vi "WILT.vi"() -> ()   [LabVIEW 2016] (continued)
        n1516 = call "WILT Station Controller.vi"("Station Number"=w3052, "GUI Aisle in"=w3054, "Drying Time (Min)"=w3037, "Current Threshold"=w3042, "Station Test State In"=w3047, "Error In"=w3051, "Aisle Location Index"=w3049, "Cool Down Period (seconds)"=w3038, "Disable Flood Check"=w3032, "Delay After Cutout (sec)"=w3034, "Previous Run Statistics"=w3036, "Send Restart Every? (Sec)"=w3039, "Agilent Valve and Switch Locations"=w3043, "Injection Times"=w3044, "Enable Start Retry"=w3041, "Day/Night Cycle"=w3045, "Final Start Presses"=w3033, "Semaphore"=w3035) -> ("GUI Aisle 1"=w3053:T3[], "Test Station Out"=w3048:T7, "Enable Start Retry Out"=w3040:bool[], "Error Out"=w3050:errorcluster)  [unwired: 5 in, 1 out]
        n1517 = Bundle By Name(cluster=w3056, "GUI Aisle 1 (SLAT)."=w3053, "Station Test State Cluster"=w3048, "Enable Start Retry Array"=w3040) -> (w3055:T24)
        n1518 = call <vilib>:"Add State(s) to Queue__jki_lib_state_machine.vi"("State(s) in (\"\")"=w3058) -> ("States Out"=w3057:string)  [unwired: 14 in]
      }
      frame "Station 12" {
        w3076 = 11  # Aisle Location Index
        w3079 = u32 12  # Station Number
        # "Control the state of station 12"
        n1519 = Unbundle By Name(w3083) -> ("Enable Start Retry Array"=w3067:bool[], "Agilent Switches"=w3069:T2[], "GUI Aisle 1 (SLAT)."=w3081:T3[], "Drying Time (Min)"=w3064:dbl[], "Current Threshold"=w3070:dbl, "Station Test State Cluster"=w3074:T7, "Station Timeout Values (1-56) Seconds"=w3065:dbl[], "Send Restart Every? (Sec)"=w3066:dbl, "Injection Times Input"=w3071:T15, "Day/Night Cycle Input"=w3072:T11)
        n1520 = local read "Previous Run Statistics"() -> (w3063:T9[])
        n1521 = local read "Delay After Cutout (Sec)"() -> (w3061:dbl)
        n1522 = local read "Final Start Presses"() -> (w3060:i32)
        n1523 = local read "Agilent Semaphore"() -> (w3062:T1[])
        n1524 = local read "Disable Flood Check"() -> (w3059:bool)
        n1525 = call "WILT Station Controller.vi"("Station Number"=w3079, "GUI Aisle in"=w3081, "Drying Time (Min)"=w3064, "Current Threshold"=w3070, "Station Test State In"=w3074, "Error In"=w3078, "Aisle Location Index"=w3076, "Cool Down Period (seconds)"=w3065, "Disable Flood Check"=w3059, "Delay After Cutout (sec)"=w3061, "Previous Run Statistics"=w3063, "Send Restart Every? (Sec)"=w3066, "Agilent Valve and Switch Locations"=w3069, "Injection Times"=w3071, "Enable Start Retry"=w3067, "Day/Night Cycle"=w3072, "Final Start Presses"=w3060, "Semaphore"=w3062) -> ("GUI Aisle 1"=w3080:T3[], "Test Station Out"=w3075:T7, "Enable Start Retry Out"=w3068:bool[], "Error Out"=w3077:errorcluster)  [unwired: 5 in, 1 out]
        n1526 = Bundle By Name(cluster=w3083, "GUI Aisle 1 (SLAT)."=w3080, "Station Test State Cluster"=w3075, "Enable Start Retry Array"=w3068) -> (w3082:T24)
        n1527 = call <vilib>:"Add State(s) to Queue__jki_lib_state_machine.vi"("State(s) in (\"\")"=w3085) -> ("States Out"=w3084:string)  [unwired: 14 in]
      }
      frame "Station 13" {
        w3104 = 0  # Aisle Location Index
        w3107 = u32 13  # Station Number
        # "Control the state of station 13"
        n1528 = Unbundle By Name(w3110) -> ("Enable Start Retry Array"=w3094:bool[], "Agilent Switches"=w3098:T2[], "GUI Aisle 1A (SLAT)."=w3108:T3[], "Drying Time (Min)"=w3091:dbl[], "Current Threshold"=w3097:dbl, "Station Test State Cluster"=w3102:T7, "Station Timeout Values (1-56) Seconds"=w3092:dbl[], "Send Restart Every? (Sec)"=w3093:dbl, "Injection Times Input"=w3099:T15, "Day/Night Cycle Input"=w3100:T11)
        n1529 = local read "Delay After Cutout (Sec)"() -> (w3088:dbl)
        n1530 = local read "Final Start Presses"() -> (w3087:i32)
        n1531 = local read "Agilent Semaphore"() -> (w3089:T1[])
        n1532 = local read "Previous Run Statistics"() -> (w3090:T9[])
        n1533 = local read "Disable Flood Check"() -> (w3086:bool)
        n1534 = call "WILT Station Controller.vi"("Station Number"=w3107, "GUI Aisle in"=w3108, "Drying Time (Min)"=w3091, "Current Threshold"=w3097, "Station Test State In"=w3102, "Error In"=w3106, "Aisle Location Index"=w3104, "Cool Down Period (seconds)"=w3092, "Disable Flood Check"=w3086, "Delay After Cutout (sec)"=w3088, "Previous Run Statistics"=w3090, "Send Restart Every? (Sec)"=w3093, "Agilent Valve and Switch Locations"=w3098, "Injection Times"=w3099, "Enable Start Retry"=w3094, "Day/Night Cycle"=w3100, "Final Start Presses"=w3087, "Semaphore"=w3089) -> ("GUI Aisle 1"=w3096:T3[], "Test Station Out"=w3103:T7, "Enable Start Retry Out"=w3095:bool[], "Error Out"=w3105:errorcluster)  [unwired: 5 in, 1 out]
        n1535 = Bundle By Name(cluster=w3110, "GUI Aisle 1A (SLAT)."=w3096, "Station Test State Cluster"=w3103, "Enable Start Retry Array"=w3095) -> (w3109:T24)
        n1536 = call <vilib>:"Add State(s) to Queue__jki_lib_state_machine.vi"("State(s) in (\"\")"=w3112) -> ("States Out"=w3111:string)  [unwired: 14 in]
      }
      frame "Station 14" {
        w3130 = 1  # Aisle Location Index
        w3133 = u32 14  # Station Number
        # "Control the state of station 14"
        n1537 = Unbundle By Name(w3137) -> ("Enable Start Retry Array"=w3122:bool[], "Agilent Switches"=w3124:T2[], "GUI Aisle 1A (SLAT)."=w3135:T3[], "Drying Time (Min)"=w3118:dbl[], "Current Threshold"=w3123:dbl, "Station Test State Cluster"=w3128:T7, "Station Timeout Values (1-56) Seconds"=w3119:dbl[], "Send Restart Every? (Sec)"=w3120:dbl, "Injection Times Input"=w3125:T15, "Day/Night Cycle Input"=w3126:T11)
        n1538 = local read "Previous Run Statistics"() -> (w3117:T9[])
        n1539 = local read "Disable Flood Check"() -> (w3113:bool)
        n1540 = local read "Delay After Cutout (Sec)"() -> (w3115:dbl)
        n1541 = local read "Final Start Presses"() -> (w3114:i32)
        n1542 = local read "Agilent Semaphore"() -> (w3116:T1[])
        n1543 = call "WILT Station Controller.vi"("Station Number"=w3133, "GUI Aisle in"=w3135, "Drying Time (Min)"=w3118, "Current Threshold"=w3123, "Station Test State In"=w3128, "Error In"=w3132, "Aisle Location Index"=w3130, "Cool Down Period (seconds)"=w3119, "Disable Flood Check"=w3113, "Delay After Cutout (sec)"=w3115, "Previous Run Statistics"=w3117, "Send Restart Every? (Sec)"=w3120, "Agilent Valve and Switch Locations"=w3124, "Injection Times"=w3125, "Enable Start Retry"=w3122, "Day/Night Cycle"=w3126, "Final Start Presses"=w3114, "Semaphore"=w3116) -> ("GUI Aisle 1"=w3134:T3[], "Test Station Out"=w3129:T7, "Enable Start Retry Out"=w3121:bool[], "Error Out"=w3131:errorcluster)  [unwired: 5 in, 1 out]
        n1544 = Bundle By Name(cluster=w3137, "GUI Aisle 1A (SLAT)."=w3134, "Station Test State Cluster"=w3129, "Enable Start Retry Array"=w3121) -> (w3136:T24)
        n1545 = call <vilib>:"Add State(s) to Queue__jki_lib_state_machine.vi"("State(s) in (\"\")"=w3139) -> ("States Out"=w3138:string)  [unwired: 14 in]
      }
      frame "Station 15" {
        w3157 = 2  # Aisle Location Index
        w3160 = u32 15  # Station Number
        # "Control the state of station 15"
        n1546 = Unbundle By Name(w3164) -> ("Enable Start Retry Array"=w3148:bool[], "Agilent Switches"=w3151:T2[], "GUI Aisle 1A (SLAT)."=w3162:T3[], "Drying Time (Min)"=w3144:dbl[], "Current Threshold"=w3150:dbl, "Station Test State Cluster"=w3155:T7, "Station Timeout Values (1-56) Seconds"=w3145:dbl[], "Send Restart Every? (Sec)"=w3147:dbl, "Injection Times Input"=w3152:T15, "Day/Night Cycle Input"=w3153:T11)
        n1547 = local read "Previous Run Statistics"() -> (w3146:T9[])
        n1548 = local read "Disable Flood Check"() -> (w3140:bool)
        n1549 = local read "Delay After Cutout (Sec)"() -> (w3142:dbl)
        n1550 = local read "Agilent Semaphore"() -> (w3143:T1[])
        n1551 = local read "Final Start Presses"() -> (w3141:i32)
        n1552 = call "WILT Station Controller.vi"("Station Number"=w3160, "GUI Aisle in"=w3162, "Drying Time (Min)"=w3144, "Current Threshold"=w3150, "Station Test State In"=w3155, "Error In"=w3159, "Aisle Location Index"=w3157, "Cool Down Period (seconds)"=w3145, "Disable Flood Check"=w3140, "Delay After Cutout (sec)"=w3142, "Previous Run Statistics"=w3146, "Send Restart Every? (Sec)"=w3147, "Agilent Valve and Switch Locations"=w3151, "Injection Times"=w3152, "Enable Start Retry"=w3148, "Day/Night Cycle"=w3153, "Final Start Presses"=w3141, "Semaphore"=w3143) -> ("GUI Aisle 1"=w3161:T3[], "Test Station Out"=w3156:T7, "Enable Start Retry Out"=w3149:bool[], "Error Out"=w3158:errorcluster)  [unwired: 5 in, 1 out]
        n1553 = Bundle By Name(cluster=w3164, "GUI Aisle 1A (SLAT)."=w3161, "Station Test State Cluster"=w3156, "Enable Start Retry Array"=w3149) -> (w3163:T24)
        n1554 = call <vilib>:"Add State(s) to Queue__jki_lib_state_machine.vi"("State(s) in (\"\")"=w3166) -> ("States Out"=w3165:string)  [unwired: 14 in]
      }
      frame "Station 16" {
        w3184 = 3  # Aisle Location Index
        w3187 = u32 16  # Station Number
        # "Control the state of station 16"
        n1555 = Unbundle By Name(w3191) -> ("Enable Start Retry Array"=w3175:bool[], "Agilent Switches"=w3177:T2[], "GUI Aisle 1A (SLAT)."=w3189:T3[], "Drying Time (Min)"=w3171:dbl[], "Current Threshold"=w3178:dbl, "Station Test State Cluster"=w3182:T7, "Station Timeout Values (1-56) Seconds"=w3172:dbl[], "Send Restart Every? (Sec)"=w3174:dbl, "Injection Times Input"=w3179:T15, "Day/Night Cycle Input"=w3180:T11)
        n1556 = local read "Previous Run Statistics"() -> (w3173:T9[])
        n1557 = local read "Disable Flood Check"() -> (w3167:bool)
        n1558 = local read "Delay After Cutout (Sec)"() -> (w3169:dbl)
        n1559 = local read "Agilent Semaphore"() -> (w3170:T1[])
        n1560 = local read "Final Start Presses"() -> (w3168:i32)
        n1561 = call "WILT Station Controller.vi"("Station Number"=w3187, "GUI Aisle in"=w3189, "Drying Time (Min)"=w3171, "Current Threshold"=w3178, "Station Test State In"=w3182, "Error In"=w3186, "Aisle Location Index"=w3184, "Cool Down Period (seconds)"=w3172, "Disable Flood Check"=w3167, "Delay After Cutout (sec)"=w3169, "Previous Run Statistics"=w3173, "Send Restart Every? (Sec)"=w3174, "Agilent Valve and Switch Locations"=w3177, "Injection Times"=w3179, "Enable Start Retry"=w3175, "Day/Night Cycle"=w3180, "Final Start Presses"=w3168, "Semaphore"=w3170) -> ("GUI Aisle 1"=w3188:T3[], "Test Station Out"=w3183:T7, "Enable Start Retry Out"=w3176:bool[], "Error Out"=w3185:errorcluster)  [unwired: 5 in, 1 out]
        n1562 = Bundle By Name(cluster=w3191, "GUI Aisle 1A (SLAT)."=w3188, "Station Test State Cluster"=w3183, "Enable Start Retry Array"=w3176) -> (w3190:T24)
        n1563 = call <vilib>:"Add State(s) to Queue__jki_lib_state_machine.vi"("State(s) in (\"\")"=w3193) -> ("States Out"=w3192:string)  [unwired: 14 in]
      }
      frame "Station 17" {
        w3211 = 4  # Aisle Location Index
        w3214 = u32 17  # Station Number
        # "Control the state of station 17"
        n1564 = Unbundle By Name(w3218) -> ("Enable Start Retry Array"=w3202:bool[], "Agilent Switches"=w3204:T2[], "GUI Aisle 1A (SLAT)."=w3216:T3[], "Drying Time (Min)"=w3198:dbl[], "Current Threshold"=w3205:dbl, "Station Test State Cluster"=w3209:T7, "Station Timeout Values (1-56) Seconds"=w3199:dbl[], "Send Restart Every? (Sec)"=w3201:dbl, "Injection Times Input"=w3206:T15, "Day/Night Cycle Input"=w3207:T11)
        n1565 = local read "Previous Run Statistics"() -> (w3200:T9[])
        n1566 = local read "Disable Flood Check"() -> (w3194:bool)
        n1567 = local read "Delay After Cutout (Sec)"() -> (w3196:dbl)
        n1568 = local read "Final Start Presses"() -> (w3195:i32)
        n1569 = local read "Agilent Semaphore"() -> (w3197:T1[])
        n1570 = call "WILT Station Controller.vi"("Station Number"=w3214, "GUI Aisle in"=w3216, "Drying Time (Min)"=w3198, "Current Threshold"=w3205, "Station Test State In"=w3209, "Error In"=w3213, "Aisle Location Index"=w3211, "Cool Down Period (seconds)"=w3199, "Disable Flood Check"=w3194, "Delay After Cutout (sec)"=w3196, "Previous Run Statistics"=w3200, "Send Restart Every? (Sec)"=w3201, "Agilent Valve and Switch Locations"=w3204, "Injection Times"=w3206, "Enable Start Retry"=w3202, "Day/Night Cycle"=w3207, "Final Start Presses"=w3195, "Semaphore"=w3197) -> ("GUI Aisle 1"=w3215:T3[], "Test Station Out"=w3210:T7, "Enable Start Retry Out"=w3203:bool[], "Error Out"=w3212:errorcluster)  [unwired: 5 in, 1 out]
        n1571 = Bundle By Name(cluster=w3218, "GUI Aisle 1A (SLAT)."=w3215, "Station Test State Cluster"=w3210, "Enable Start Retry Array"=w3203) -> (w3217:T24)
        n1572 = call <vilib>:"Add State(s) to Queue__jki_lib_state_machine.vi"("State(s) in (\"\")"=w3220) -> ("States Out"=w3219:string)  [unwired: 14 in]
      }
      frame "Station 18" {
        w3238 = 5  # Aisle Location Index
        w3241 = u32 18  # Station Number
        # "Control the state of station 18"
        n1573 = Unbundle By Name(w3245) -> ("Enable Start Retry Array"=w3229:bool[], "Agilent Switches"=w3231:T2[], "GUI Aisle 1A (SLAT)."=w3243:T3[], "Drying Time (Min)"=w3225:dbl[], "Current Threshold"=w3232:dbl, "Station Test State Cluster"=w3236:T7, "Station Timeout Values (1-56) Seconds"=w3226:dbl[], "Send Restart Every? (Sec)"=w3228:dbl, "Injection Times Input"=w3233:T15, "Day/Night Cycle Input"=w3234:T11)
        n1574 = local read "Delay After Cutout (Sec)"() -> (w3223:dbl)
        n1575 = local read "Final Start Presses"() -> (w3222:i32)
        n1576 = local read "Agilent Semaphore"() -> (w3224:T1[])
        n1577 = local read "Previous Run Statistics"() -> (w3227:T9[])
        n1578 = local read "Disable Flood Check"() -> (w3221:bool)
        n1579 = call "WILT Station Controller.vi"("Station Number"=w3241, "GUI Aisle in"=w3243, "Drying Time (Min)"=w3225, "Current Threshold"=w3232, "Station Test State In"=w3236, "Error In"=w3240, "Aisle Location Index"=w3238, "Cool Down Period (seconds)"=w3226, "Disable Flood Check"=w3221, "Delay After Cutout (sec)"=w3223, "Previous Run Statistics"=w3227, "Send Restart Every? (Sec)"=w3228, "Agilent Valve and Switch Locations"=w3231, "Injection Times"=w3233, "Enable Start Retry"=w3229, "Day/Night Cycle"=w3234, "Final Start Presses"=w3222, "Semaphore"=w3224) -> ("GUI Aisle 1"=w3242:T3[], "Test Station Out"=w3237:T7, "Enable Start Retry Out"=w3230:bool[], "Error Out"=w3239:errorcluster)  [unwired: 5 in, 1 out]
        n1580 = Bundle By Name(cluster=w3245, "GUI Aisle 1A (SLAT)."=w3242, "Station Test State Cluster"=w3237, "Enable Start Retry Array"=w3230) -> (w3244:T24)
        n1581 = call <vilib>:"Add State(s) to Queue__jki_lib_state_machine.vi"("State(s) in (\"\")"=w3247) -> ("States Out"=w3246:string)  [unwired: 14 in]
      }
      frame "Station 19" {
        w3265 = 6  # Aisle Location Index
        w3268 = u32 19  # Station Number
        # "Control the state of station 19"
        n1582 = Unbundle By Name(w3272) -> ("Enable Start Retry Array"=w3256:bool[], "Agilent Switches"=w3259:T2[], "GUI Aisle 1A (SLAT)."=w3270:T3[], "Drying Time (Min)"=w3252:dbl[], "Current Threshold"=w3258:dbl, "Station Test State Cluster"=w3263:T7, "Station Timeout Values (1-56) Seconds"=w3253:dbl[], "Send Restart Every? (Sec)"=w3255:dbl, "Injection Times Input"=w3260:T15, "Day/Night Cycle Input"=w3261:T11)
        n1583 = local read "Delay After Cutout (Sec)"() -> (w3250:dbl)
        n1584 = local read "Final Start Presses"() -> (w3249:i32)
        n1585 = local read "Agilent Semaphore"() -> (w3251:T1[])
        n1586 = local read "Previous Run Statistics"() -> (w3254:T9[])
        n1587 = local read "Disable Flood Check"() -> (w3248:bool)
        n1588 = call "WILT Station Controller.vi"("Station Number"=w3268, "GUI Aisle in"=w3270, "Drying Time (Min)"=w3252, "Current Threshold"=w3258, "Station Test State In"=w3263, "Error In"=w3267, "Aisle Location Index"=w3265, "Cool Down Period (seconds)"=w3253, "Disable Flood Check"=w3248, "Delay After Cutout (sec)"=w3250, "Previous Run Statistics"=w3254, "Send Restart Every? (Sec)"=w3255, "Agilent Valve and Switch Locations"=w3259, "Injection Times"=w3260, "Enable Start Retry"=w3256, "Day/Night Cycle"=w3261, "Final Start Presses"=w3249, "Semaphore"=w3251) -> ("GUI Aisle 1"=w3269:T3[], "Test Station Out"=w3264:T7, "Enable Start Retry Out"=w3257:bool[], "Error Out"=w3266:errorcluster)  [unwired: 5 in, 1 out]
        n1589 = Bundle By Name(cluster=w3272, "GUI Aisle 1A (SLAT)."=w3269, "Station Test State Cluster"=w3264, "Enable Start Retry Array"=w3257) -> (w3271:T24)
        n1590 = call <vilib>:"Add State(s) to Queue__jki_lib_state_machine.vi"("State(s) in (\"\")"=w3274) -> ("States Out"=w3273:string)  [unwired: 14 in]
      }
      frame "Station 20" {
        w3292 = 7  # Aisle Location Index
        w3295 = u32 20  # Station Number
        # "Control the state of station 20"
        n1591 = Unbundle By Name(w3299) -> ("Enable Start Retry Array"=w3283:bool[], "Agilent Switches"=w3286:T2[], "GUI Aisle 1A (SLAT)."=w3297:T3[], "Drying Time (Min)"=w3279:dbl[], "Current Threshold"=w3285:dbl, "Station Test State Cluster"=w3290:T7, "Station Timeout Values (1-56) Seconds"=w3280:dbl[], "Send Restart Every? (Sec)"=w3282:dbl, "Injection Times Input"=w3287:T15, "Day/Night Cycle Input"=w3288:T11)
        n1592 = local read "Previous Run Statistics"() -> (w3281:T9[])
        n1593 = local read "Delay After Cutout (Sec)"() -> (w3277:dbl)
        n1594 = local read "Final Start Presses"() -> (w3276:i32)
        n1595 = local read "Agilent Semaphore"() -> (w3278:T1[])
        n1596 = local read "Disable Flood Check"() -> (w3275:bool)
        n1597 = call "WILT Station Controller.vi"("Station Number"=w3295, "GUI Aisle in"=w3297, "Drying Time (Min)"=w3279, "Current Threshold"=w3285, "Station Test State In"=w3290, "Error In"=w3294, "Aisle Location Index"=w3292, "Cool Down Period (seconds)"=w3280, "Disable Flood Check"=w3275, "Delay After Cutout (sec)"=w3277, "Previous Run Statistics"=w3281, "Send Restart Every? (Sec)"=w3282, "Agilent Valve and Switch Locations"=w3286, "Injection Times"=w3287, "Enable Start Retry"=w3283, "Day/Night Cycle"=w3288, "Final Start Presses"=w3276, "Semaphore"=w3278) -> ("GUI Aisle 1"=w3296:T3[], "Test Station Out"=w3291:T7, "Enable Start Retry Out"=w3284:bool[], "Error Out"=w3293:errorcluster)  [unwired: 5 in, 1 out]
        n1598 = Bundle By Name(cluster=w3299, "GUI Aisle 1A (SLAT)."=w3296, "Station Test State Cluster"=w3291, "Enable Start Retry Array"=w3284) -> (w3298:T24)
        n1599 = call <vilib>:"Add State(s) to Queue__jki_lib_state_machine.vi"("State(s) in (\"\")"=w3301) -> ("States Out"=w3300:string)  [unwired: 14 in]
      }
      frame "Station 21" {
        w3319 = 0  # Aisle Location Index
        w3322 = u32 21  # Station Number
        # "Control the state of station 21"
        n1600 = Unbundle By Name(w3326) -> ("Enable Start Retry Array"=w3310:bool[], "Agilent Switches"=w3312:T2[], "GUI Aisle 2."=w3324:T3[], "Drying Time (Min)"=w3306:dbl[], "Current Threshold"=w3313:dbl, "Station Test State Cluster"=w3317:T7, "Station Timeout Values (1-56) Seconds"=w3307:dbl[], "Send Restart Every? (Sec)"=w3309:dbl, "Injection Times Input"=w3314:T15, "Day/Night Cycle Input"=w3315:T11)
        n1601 = local read "Delay After Cutout (Sec)"() -> (w3304:dbl)
        n1602 = local read "Agilent Semaphore"() -> (w3305:T1[])
        n1603 = local read "Final Start Presses"() -> (w3303:i32)
        n1604 = local read "Previous Run Statistics"() -> (w3308:T9[])
        n1605 = local read "Disable Flood Check"() -> (w3302:bool)
        n1606 = call "WILT Station Controller.vi"("Station Number"=w3322, "GUI Aisle in"=w3324, "Drying Time (Min)"=w3306, "Current Threshold"=w3313, "Station Test State In"=w3317, "Error In"=w3321, "Aisle Location Index"=w3319, "Cool Down Period (seconds)"=w3307, "Disable Flood Check"=w3302, "Delay After Cutout (sec)"=w3304, "Previous Run Statistics"=w3308, "Send Restart Every? (Sec)"=w3309, "Agilent Valve and Switch Locations"=w3312, "Injection Times"=w3314, "Enable Start Retry"=w3310, "Day/Night Cycle"=w3315, "Final Start Presses"=w3303, "Semaphore"=w3305) -> ("GUI Aisle 1"=w3323:T3[], "Test Station Out"=w3318:T7, "Enable Start Retry Out"=w3311:bool[], "Error Out"=w3320:errorcluster)  [unwired: 5 in, 1 out]
        n1607 = call <vilib>:"Add State(s) to Queue__jki_lib_state_machine.vi"("State(s) in (\"\")"=w3328) -> ("States Out"=w3327:string)  [unwired: 14 in]
        n1608 = Bundle By Name(cluster=w3326, "GUI Aisle 2."=w3323, "Station Test State Cluster"=w3318, "Enable Start Retry Array"=w3311) -> (w3325:T24)
      }
      frame "Station 22" {
        w3346 = 1  # Aisle Location Index
        w3349 = u32 22  # Station Number
        # "Control the state of station 22"
        n1609 = Unbundle By Name(w3353) -> ("Enable Start Retry Array"=w3337:bool[], "Agilent Switches"=w3340:T2[], "GUI Aisle 2."=w3351:T3[], "Drying Time (Min)"=w3333:dbl[], "Current Threshold"=w3339:dbl, "Station Test State Cluster"=w3345:T7, "Station Timeout Values (1-56) Seconds"=w3334:dbl[], "Send Restart Every? (Sec)"=w3336:dbl, "Injection Times Input"=w3341:T15, "Day/Night Cycle Input"=w3342:T11)
        n1610 = local read "Previous Run Statistics"() -> (w3335:T9[])
        n1611 = local read "Disable Flood Check"() -> (w3329:bool)
        n1612 = local read "Delay After Cutout (Sec)"() -> (w3331:dbl)
        n1613 = local read "Final Start Presses"() -> (w3330:i32)
        n1614 = local read "Agilent Semaphore"() -> (w3332:T1[])
        n1615 = call "WILT Station Controller.vi"("Station Number"=w3349, "GUI Aisle in"=w3351, "Drying Time (Min)"=w3333, "Current Threshold"=w3339, "Station Test State In"=w3345, "Error In"=w3348, "Aisle Location Index"=w3346, "Cool Down Period (seconds)"=w3334, "Disable Flood Check"=w3329, "Delay After Cutout (sec)"=w3331, "Previous Run Statistics"=w3335, "Send Restart Every? (Sec)"=w3336, "Agilent Valve and Switch Locations"=w3340, "Injection Times"=w3341, "Enable Start Retry"=w3337, "Day/Night Cycle"=w3342, "Final Start Presses"=w3330, "Semaphore"=w3332) -> ("GUI Aisle 1"=w3350:T3[], "Test Station Out"=w3344:T7, "Enable Start Retry Out"=w3338:bool[], "Error Out"=w3347:errorcluster)  [unwired: 5 in, 1 out]
        n1616 = Bundle By Name(cluster=w3353, "GUI Aisle 2."=w3350, "Station Test State Cluster"=w3344, "Enable Start Retry Array"=w3338) -> (w3352:T24)
        n1617 = call <vilib>:"Add State(s) to Queue__jki_lib_state_machine.vi"("State(s) in (\"\")"=w3355) -> ("States Out"=w3354:string)  [unwired: 14 in]
      }
      frame "Station 23" {
        w3373 = 2  # Aisle Location Index
        w3376 = u32 23  # Station Number
        # "Control the state of station 23"
        n1618 = Unbundle By Name(w3380) -> ("Enable Start Retry Array"=w3364:bool[], "Agilent Switches"=w3367:T2[], "GUI Aisle 2."=w3378:T3[], "Drying Time (Min)"=w3360:dbl[], "Current Threshold"=w3366:dbl, "Station Test State Cluster"=w3371:T7, "Station Timeout Values (1-56) Seconds"=w3361:dbl[], "Send Restart Every? (Sec)"=w3363:dbl, "Injection Times Input"=w3368:T15, "Day/Night Cycle Input"=w3369:T11)
        n1619 = local read "Delay After Cutout (Sec)"() -> (w3358:dbl)
        n1620 = local read "Final Start Presses"() -> (w3357:i32)
        n1621 = local read "Agilent Semaphore"() -> (w3359:T1[])
        n1622 = local read "Previous Run Statistics"() -> (w3362:T9[])
        n1623 = local read "Disable Flood Check"() -> (w3356:bool)
        n1624 = call "WILT Station Controller.vi"("Station Number"=w3376, "GUI Aisle in"=w3378, "Drying Time (Min)"=w3360, "Current Threshold"=w3366, "Station Test State In"=w3371, "Error In"=w3375, "Aisle Location Index"=w3373, "Cool Down Period (seconds)"=w3361, "Disable Flood Check"=w3356, "Delay After Cutout (sec)"=w3358, "Previous Run Statistics"=w3362, "Send Restart Every? (Sec)"=w3363, "Agilent Valve and Switch Locations"=w3367, "Injection Times"=w3368, "Enable Start Retry"=w3364, "Day/Night Cycle"=w3369, "Final Start Presses"=w3357, "Semaphore"=w3359) -> ("GUI Aisle 1"=w3377:T3[], "Test Station Out"=w3372:T7, "Enable Start Retry Out"=w3365:bool[], "Error Out"=w3374:errorcluster)  [unwired: 5 in, 1 out]
        n1625 = Bundle By Name(cluster=w3380, "GUI Aisle 2."=w3377, "Station Test State Cluster"=w3372, "Enable Start Retry Array"=w3365) -> (w3379:T24)
        n1626 = call <vilib>:"Add State(s) to Queue__jki_lib_state_machine.vi"("State(s) in (\"\")"=w3382) -> ("States Out"=w3381:string)  [unwired: 14 in]
      }
      frame "Station 24" {
        w3400 = 3  # Aisle Location Index
        w3403 = u32 24  # Station Number
        # "Control the state of station 24"
        n1627 = Unbundle By Name(w3407) -> ("Enable Start Retry Array"=w3392:bool[], "Agilent Switches"=w3394:T2[], "GUI Aisle 2."=w3405:T3[], "Drying Time (Min)"=w3387:dbl[], "Current Threshold"=w3393:dbl, "Station Test State Cluster"=w3398:T7, "Station Timeout Values (1-56) Seconds"=w3388:dbl[], "Send Restart Every? (Sec)"=w3390:dbl, "Injection Times Input"=w3395:T15, "Day/Night Cycle Input"=w3396:T11)
        n1628 = local read "Previous Run Statistics"() -> (w3389:T9[])
        n1629 = local read "Disable Flood Check"() -> (w3383:bool)
        n1630 = local read "Delay After Cutout (Sec)"() -> (w3385:dbl)
        n1631 = local read "Final Start Presses"() -> (w3384:i32)
        n1632 = local read "Agilent Semaphore"() -> (w3386:T1[])
        n1633 = call "WILT Station Controller.vi"("Station Number"=w3403, "GUI Aisle in"=w3405, "Drying Time (Min)"=w3387, "Current Threshold"=w3393, "Station Test State In"=w3398, "Error In"=w3402, "Aisle Location Index"=w3400, "Cool Down Period (seconds)"=w3388, "Disable Flood Check"=w3383, "Delay After Cutout (sec)"=w3385, "Previous Run Statistics"=w3389, "Send Restart Every? (Sec)"=w3390, "Agilent Valve and Switch Locations"=w3394, "Injection Times"=w3395, "Enable Start Retry"=w3392, "Day/Night Cycle"=w3396, "Final Start Presses"=w3384, "Semaphore"=w3386) -> ("GUI Aisle 1"=w3404:T3[], "Test Station Out"=w3399:T7, "Enable Start Retry Out"=w3391:bool[], "Error Out"=w3401:errorcluster)  [unwired: 5 in, 1 out]
        n1634 = Bundle By Name(cluster=w3407, "GUI Aisle 2."=w3404, "Station Test State Cluster"=w3399, "Enable Start Retry Array"=w3391) -> (w3406:T24)
        n1635 = call <vilib>:"Add State(s) to Queue__jki_lib_state_machine.vi"("State(s) in (\"\")"=w3409) -> ("States Out"=w3408:string)  [unwired: 14 in]
      }
      frame "Station 25" {
        w3427 = 4  # Aisle Location Index
        w3430 = u32 25  # Station Number
        # "Control the state of station 25"
        n1636 = Unbundle By Name(w3434) -> ("Enable Start Retry Array"=w3418:bool[], "Agilent Switches"=w3421:T2[], "GUI Aisle 2."=w3432:T3[], "Drying Time (Min)"=w3414:dbl[], "Current Threshold"=w3420:dbl, "Station Test State Cluster"=w3425:T7, "Station Timeout Values (1-56) Seconds"=w3415:dbl[], "Send Restart Every? (Sec)"=w3417:dbl, "Injection Times Input"=w3422:T15, "Day/Night Cycle Input"=w3423:T11)
        n1637 = local read "Delay After Cutout (Sec)"() -> (w3412:dbl)
        n1638 = local read "Final Start Presses"() -> (w3411:i32)
        n1639 = local read "Agilent Semaphore"() -> (w3413:T1[])
        n1640 = local read "Previous Run Statistics"() -> (w3416:T9[])
        n1641 = local read "Disable Flood Check"() -> (w3410:bool)
        n1642 = call "WILT Station Controller.vi"("Station Number"=w3430, "GUI Aisle in"=w3432, "Drying Time (Min)"=w3414, "Current Threshold"=w3420, "Station Test State In"=w3425, "Error In"=w3429, "Aisle Location Index"=w3427, "Cool Down Period (seconds)"=w3415, "Disable Flood Check"=w3410, "Delay After Cutout (sec)"=w3412, "Previous Run Statistics"=w3416, "Send Restart Every? (Sec)"=w3417, "Agilent Valve and Switch Locations"=w3421, "Injection Times"=w3422, "Enable Start Retry"=w3418, "Day/Night Cycle"=w3423, "Final Start Presses"=w3411, "Semaphore"=w3413) -> ("GUI Aisle 1"=w3431:T3[], "Test Station Out"=w3426:T7, "Enable Start Retry Out"=w3419:bool[], "Error Out"=w3428:errorcluster)  [unwired: 5 in, 1 out]
        n1643 = Bundle By Name(cluster=w3434, "GUI Aisle 2."=w3431, "Station Test State Cluster"=w3426, "Enable Start Retry Array"=w3419) -> (w3433:T24)
        n1644 = call <vilib>:"Add State(s) to Queue__jki_lib_state_machine.vi"("State(s) in (\"\")"=w3436) -> ("States Out"=w3435:string)  [unwired: 14 in]
      }
      frame "Station 26" {
        w3454 = 5  # Aisle Location Index
        w3457 = u32 26  # Station Number
        # "Control the state of station 26"
        n1645 = Unbundle By Name(w3461) -> ("Enable Start Retry Array"=w3445:bool[], "Agilent Switches"=w3449:T2[], "GUI Aisle 2."=w3459:T3[], "Drying Time (Min)"=w3441:dbl[], "Current Threshold"=w3448:dbl, "Station Test State Cluster"=w3452:T7, "Station Timeout Values (1-56) Seconds"=w3442:dbl[], "Send Restart Every? (Sec)"=w3444:dbl, "Injection Times Input"=w3450:T15, "Day/Night Cycle Input"=w3447:T11)
        n1646 = local read "Delay After Cutout (Sec)"() -> (w3439:dbl)
        n1647 = local read "Final Start Presses"() -> (w3438:i32)
        n1648 = local read "Agilent Semaphore"() -> (w3440:T1[])
        n1649 = local read "Previous Run Statistics"() -> (w3443:T9[])
        n1650 = local read "Disable Flood Check"() -> (w3437:bool)
        n1651 = call "WILT Station Controller.vi"("Station Number"=w3457, "GUI Aisle in"=w3459, "Drying Time (Min)"=w3441, "Current Threshold"=w3448, "Station Test State In"=w3452, "Error In"=w3456, "Aisle Location Index"=w3454, "Cool Down Period (seconds)"=w3442, "Disable Flood Check"=w3437, "Delay After Cutout (sec)"=w3439, "Previous Run Statistics"=w3443, "Send Restart Every? (Sec)"=w3444, "Agilent Valve and Switch Locations"=w3449, "Injection Times"=w3450, "Enable Start Retry"=w3445, "Day/Night Cycle"=w3447, "Final Start Presses"=w3438, "Semaphore"=w3440) -> ("GUI Aisle 1"=w3458:T3[], "Test Station Out"=w3453:T7, "Enable Start Retry Out"=w3446:bool[], "Error Out"=w3455:errorcluster)  [unwired: 5 in, 1 out]
        n1652 = Bundle By Name(cluster=w3461, "GUI Aisle 2."=w3458, "Station Test State Cluster"=w3453, "Enable Start Retry Array"=w3446) -> (w3460:T24)
        n1653 = call <vilib>:"Add State(s) to Queue__jki_lib_state_machine.vi"("State(s) in (\"\")"=w3463) -> ("States Out"=w3462:string)  [unwired: 14 in]
      }
      frame "Station 27" {
        w3481 = 6  # Aisle Location Index
        w3484 = u32 27  # Station Number
        # "Control the state of station 27"
        n1654 = Unbundle By Name(w3488) -> ("Enable Start Retry Array"=w3473:bool[], "Agilent Switches"=w3475:T2[], "GUI Aisle 2."=w3486:T3[], "Drying Time (Min)"=w3468:dbl[], "Current Threshold"=w3474:dbl, "Station Test State Cluster"=w3479:T7, "Station Timeout Values (1-56) Seconds"=w3469:dbl[], "Send Restart Every? (Sec)"=w3471:dbl, "Injection Times Input"=w3476:T15, "Day/Night Cycle Input"=w3477:T11)
        n1655 = local read "Delay After Cutout (Sec)"() -> (w3466:dbl)
        n1656 = local read "Final Start Presses"() -> (w3465:i32)
        n1657 = local read "Agilent Semaphore"() -> (w3467:T1[])
        n1658 = local read "Previous Run Statistics"() -> (w3470:T9[])
        n1659 = local read "Disable Flood Check"() -> (w3464:bool)
        n1660 = call "WILT Station Controller.vi"("Station Number"=w3484, "GUI Aisle in"=w3486, "Drying Time (Min)"=w3468, "Current Threshold"=w3474, "Station Test State In"=w3479, "Error In"=w3483, "Aisle Location Index"=w3481, "Cool Down Period (seconds)"=w3469, "Disable Flood Check"=w3464, "Delay After Cutout (sec)"=w3466, "Previous Run Statistics"=w3470, "Send Restart Every? (Sec)"=w3471, "Agilent Valve and Switch Locations"=w3475, "Injection Times"=w3476, "Enable Start Retry"=w3473, "Day/Night Cycle"=w3477, "Final Start Presses"=w3465, "Semaphore"=w3467) -> ("GUI Aisle 1"=w3485:T3[], "Test Station Out"=w3480:T7, "Enable Start Retry Out"=w3472:bool[], "Error Out"=w3482:errorcluster)  [unwired: 5 in, 1 out]
        n1661 = Bundle By Name(cluster=w3488, "GUI Aisle 2."=w3485, "Station Test State Cluster"=w3480, "Enable Start Retry Array"=w3472) -> (w3487:T24)
        n1662 = call <vilib>:"Add State(s) to Queue__jki_lib_state_machine.vi"("State(s) in (\"\")"=w3490) -> ("States Out"=w3489:string)  [unwired: 14 in]
      }
      frame "Station 28" {
        w3508 = 7  # Aisle Location Index
        w3511 = u32 28  # Station Number
        # "Control the state of station 28"
        n1663 = Unbundle By Name(w3515) -> ("Enable Start Retry Array"=w3500:bool[], "Agilent Switches"=w3502:T2[], "GUI Aisle 2."=w3513:T3[], "Drying Time (Min)"=w3495:dbl[], "Current Threshold"=w3501:dbl, "Station Test State Cluster"=w3506:T7, "Station Timeout Values (1-56) Seconds"=w3496:dbl[], "Send Restart Every? (Sec)"=w3498:dbl, "Injection Times Input"=w3503:T15, "Day/Night Cycle Input"=w3504:T11)
        n1664 = local read "Delay After Cutout (Sec)"() -> (w3493:dbl)
        n1665 = local read "Final Start Presses"() -> (w3492:i32)
        n1666 = local read "Agilent Semaphore"() -> (w3494:T1[])
        n1667 = local read "Previous Run Statistics"() -> (w3497:T9[])
        n1668 = local read "Disable Flood Check"() -> (w3491:bool)
        n1669 = call "WILT Station Controller.vi"("Station Number"=w3511, "GUI Aisle in"=w3513, "Drying Time (Min)"=w3495, "Current Threshold"=w3501, "Station Test State In"=w3506, "Error In"=w3510, "Aisle Location Index"=w3508, "Cool Down Period (seconds)"=w3496, "Disable Flood Check"=w3491, "Delay After Cutout (sec)"=w3493, "Previous Run Statistics"=w3497, "Send Restart Every? (Sec)"=w3498, "Agilent Valve and Switch Locations"=w3502, "Injection Times"=w3503, "Enable Start Retry"=w3500, "Day/Night Cycle"=w3504, "Final Start Presses"=w3492, "Semaphore"=w3494) -> ("GUI Aisle 1"=w3512:T3[], "Test Station Out"=w3507:T7, "Enable Start Retry Out"=w3499:bool[], "Error Out"=w3509:errorcluster)  [unwired: 5 in, 1 out]
        n1670 = Bundle By Name(cluster=w3515, "GUI Aisle 2."=w3512, "Station Test State Cluster"=w3507, "Enable Start Retry Array"=w3499) -> (w3514:T24)
        n1671 = call <vilib>:"Add State(s) to Queue__jki_lib_state_machine.vi"("State(s) in (\"\")"=w3517) -> ("States Out"=w3516:string)  [unwired: 14 in]
      }
      frame "Station 29" {
        w3535 = 8  # Aisle Location Index
        w3538 = u32 29  # Station Number
        # "Control the state of station 29"
        n1672 = Unbundle By Name(w3542) -> ("Enable Start Retry Array"=w3527:bool[], "Agilent Switches"=w3529:T2[], "GUI Aisle 2."=w3540:T3[], "Drying Time (Min)"=w3522:dbl[], "Current Threshold"=w3528:dbl, "Station Test State Cluster"=w3533:T7, "Station Timeout Values (1-56) Seconds"=w3523:dbl[], "Send Restart Every? (Sec)"=w3525:dbl, "Injection Times Input"=w3531:T15, "Day/Night Cycle Input"=w3530:T11)
        n1673 = local read "Delay After Cutout (Sec)"() -> (w3520:dbl)
        n1674 = local read "Final Start Presses"() -> (w3519:i32)
        n1675 = local read "Agilent Semaphore"() -> (w3521:T1[])
        n1676 = local read "Previous Run Statistics"() -> (w3524:T9[])
        n1677 = local read "Disable Flood Check"() -> (w3518:bool)
        n1678 = call "WILT Station Controller.vi"("Station Number"=w3538, "GUI Aisle in"=w3540, "Drying Time (Min)"=w3522, "Current Threshold"=w3528, "Station Test State In"=w3533, "Error In"=w3537, "Aisle Location Index"=w3535, "Cool Down Period (seconds)"=w3523, "Disable Flood Check"=w3518, "Delay After Cutout (sec)"=w3520, "Previous Run Statistics"=w3524, "Send Restart Every? (Sec)"=w3525, "Agilent Valve and Switch Locations"=w3529, "Injection Times"=w3531, "Enable Start Retry"=w3527, "Day/Night Cycle"=w3530, "Final Start Presses"=w3519, "Semaphore"=w3521) -> ("GUI Aisle 1"=w3539:T3[], "Test Station Out"=w3534:T7, "Enable Start Retry Out"=w3526:bool[], "Error Out"=w3536:errorcluster)  [unwired: 5 in, 1 out]
        n1679 = Bundle By Name(cluster=w3542, "GUI Aisle 2."=w3539, "Station Test State Cluster"=w3534, "Enable Start Retry Array"=w3526) -> (w3541:T24)
        n1680 = call <vilib>:"Add State(s) to Queue__jki_lib_state_machine.vi"("State(s) in (\"\")"=w3544) -> ("States Out"=w3543:string)  [unwired: 14 in]
      }
      frame "Station 30" {
        w3562 = 9  # Aisle Location Index
        w3565 = u32 30  # Station Number
        # "Control the state of station 30"
        n1681 = Unbundle By Name(w3569) -> ("Enable Start Retry Array"=w3553:bool[], "Agilent Switches"=w3556:T2[], "GUI Aisle 2."=w3567:T3[], "Drying Time (Min)"=w3549:dbl[], "Current Threshold"=w3555:dbl, "Station Test State Cluster"=w3560:T7, "Station Timeout Values (1-56) Seconds"=w3550:dbl[], "Send Restart Every? (Sec)"=w3552:dbl, "Injection Times Input"=w3558:T15, "Day/Night Cycle Input"=w3557:T11)
        n1682 = local read "Delay After Cutout (Sec)"() -> (w3547:dbl)
        n1683 = local read "Previous Run Statistics"() -> (w3551:T9[])
        n1684 = local read "Agilent Semaphore"() -> (w3548:T1[])
        n1685 = local read "Disable Flood Check"() -> (w3545:bool)
        n1686 = local read "Final Start Presses"() -> (w3546:i32)
        n1687 = call "WILT Station Controller.vi"("Station Number"=w3565, "GUI Aisle in"=w3567, "Drying Time (Min)"=w3549, "Current Threshold"=w3555, "Station Test State In"=w3560, "Error In"=w3564, "Aisle Location Index"=w3562, "Cool Down Period (seconds)"=w3550, "Disable Flood Check"=w3545, "Delay After Cutout (sec)"=w3547, "Previous Run Statistics"=w3551, "Send Restart Every? (Sec)"=w3552, "Agilent Valve and Switch Locations"=w3556, "Injection Times"=w3558, "Enable Start Retry"=w3553, "Day/Night Cycle"=w3557, "Final Start Presses"=w3546, "Semaphore"=w3548) -> ("GUI Aisle 1"=w3566:T3[], "Test Station Out"=w3561:T7, "Enable Start Retry Out"=w3554:bool[], "Error Out"=w3563:errorcluster)  [unwired: 5 in, 1 out]
        n1688 = Bundle By Name(cluster=w3569, "GUI Aisle 2."=w3566, "Station Test State Cluster"=w3561, "Enable Start Retry Array"=w3554) -> (w3568:T24)
        n1689 = call <vilib>:"Add State(s) to Queue__jki_lib_state_machine.vi"("State(s) in (\"\")"=w3571) -> ("States Out"=w3570:string)  [unwired: 14 in]
      }
      frame "Station 31" {
        w3589 = 10  # Aisle Location Index
        w3592 = u32 31  # Station Number
        # "Control the state of station 31"
        n1690 = Unbundle By Name(w3596) -> ("Enable Start Retry Array"=w3581:bool[], "Agilent Switches"=w3583:T2[], "GUI Aisle 2."=w3594:T3[], "Drying Time (Min)"=w3576:dbl[], "Current Threshold"=w3582:dbl, "Station Test State Cluster"=w3587:T7, "Station Timeout Values (1-56) Seconds"=w3577:dbl[], "Send Restart Every? (Sec)"=w3579:dbl, "Injection Times Input"=w3585:T15, "Day/Night Cycle Input"=w3584:T11)
        n1691 = local read "Delay After Cutout (Sec)"() -> (w3574:dbl)
        n1692 = local read "Final Start Presses"() -> (w3573:i32)
        n1693 = local read "Agilent Semaphore"() -> (w3575:T1[])
        n1694 = local read "Previous Run Statistics"() -> (w3578:T9[])
        n1695 = local read "Disable Flood Check"() -> (w3572:bool)
        n1696 = call "WILT Station Controller.vi"("Station Number"=w3592, "GUI Aisle in"=w3594, "Drying Time (Min)"=w3576, "Current Threshold"=w3582, "Station Test State In"=w3587, "Error In"=w3591, "Aisle Location Index"=w3589, "Cool Down Period (seconds)"=w3577, "Disable Flood Check"=w3572, "Delay After Cutout (sec)"=w3574, "Previous Run Statistics"=w3578, "Send Restart Every? (Sec)"=w3579, "Agilent Valve and Switch Locations"=w3583, "Injection Times"=w3585, "Enable Start Retry"=w3581, "Day/Night Cycle"=w3584, "Final Start Presses"=w3573, "Semaphore"=w3575) -> ("GUI Aisle 1"=w3593:T3[], "Test Station Out"=w3588:T7, "Enable Start Retry Out"=w3580:bool[], "Error Out"=w3590:errorcluster)  [unwired: 5 in, 1 out]
        n1697 = Bundle By Name(cluster=w3596, "GUI Aisle 2."=w3593, "Station Test State Cluster"=w3588, "Enable Start Retry Array"=w3580) -> (w3595:T24)
        n1698 = call <vilib>:"Add State(s) to Queue__jki_lib_state_machine.vi"("State(s) in (\"\")"=w3598) -> ("States Out"=w3597:string)  [unwired: 14 in]
      }
      frame "Station 32" {
        w3616 = 11  # Aisle Location Index
        w3619 = u32 32  # Station Number
        # "Control the state of station 32"
        n1699 = Unbundle By Name(w3623) -> ("Enable Start Retry Array"=w3608:bool[], "Agilent Switches"=w3610:T2[], "GUI Aisle 2."=w3621:T3[], "Drying Time (Min)"=w3603:dbl[], "Current Threshold"=w3609:dbl, "Station Test State Cluster"=w3614:T7, "Station Timeout Values (1-56) Seconds"=w3604:dbl[], "Send Restart Every? (Sec)"=w3606:dbl, "Injection Times Input"=w3611:T15, "Day/Night Cycle Input"=w3612:T11)
        n1700 = local read "Delay After Cutout (Sec)"() -> (w3601:dbl)
        n1701 = local read "Final Start Presses"() -> (w3600:i32)
        n1702 = local read "Agilent Semaphore"() -> (w3602:T1[])
        n1703 = local read "Previous Run Statistics"() -> (w3605:T9[])
        n1704 = local read "Disable Flood Check"() -> (w3599:bool)
        n1705 = call "WILT Station Controller.vi"("Station Number"=w3619, "GUI Aisle in"=w3621, "Drying Time (Min)"=w3603, "Current Threshold"=w3609, "Station Test State In"=w3614, "Error In"=w3618, "Aisle Location Index"=w3616, "Cool Down Period (seconds)"=w3604, "Disable Flood Check"=w3599, "Delay After Cutout (sec)"=w3601, "Previous Run Statistics"=w3605, "Send Restart Every? (Sec)"=w3606, "Agilent Valve and Switch Locations"=w3610, "Injection Times"=w3611, "Enable Start Retry"=w3608, "Day/Night Cycle"=w3612, "Final Start Presses"=w3600, "Semaphore"=w3602) -> ("GUI Aisle 1"=w3620:T3[], "Test Station Out"=w3615:T7, "Enable Start Retry Out"=w3607:bool[], "Error Out"=w3617:errorcluster)  [unwired: 5 in, 1 out]
        n1706 = Bundle By Name(cluster=w3623, "GUI Aisle 2."=w3620, "Station Test State Cluster"=w3615, "Enable Start Retry Array"=w3607) -> (w3622:T24)
        n1707 = call <vilib>:"Add State(s) to Queue__jki_lib_state_machine.vi"("State(s) in (\"\")"=w3625) -> ("States Out"=w3624:string)  [unwired: 14 in]
      }
      frame "Station 33" {
        w3643 = 0  # Aisle Location Index
        w3646 = u32 33  # Station Number
        # "Control the state of station 33"
        n1708 = Unbundle By Name(w3650) -> ("Enable Start Retry Array"=w3635:bool[], "Agilent Switches"=w3637:T2[], "GUI Aisle 3."=w3648:T3[], "Drying Time (Min)"=w3630:dbl[], "Current Threshold"=w3636:dbl, "Station Test State Cluster"=w3641:T7, "Station Timeout Values (1-56) Seconds"=w3631:dbl[], "Send Restart Every? (Sec)"=w3633:dbl, "Injection Times Input"=w3639:T15, "Day/Night Cycle Input"=w3638:T11)
        n1709 = local read "Delay After Cutout (Sec)"() -> (w3628:dbl)
        n1710 = local read "Final Start Presses"() -> (w3627:i32)
        n1711 = local read "Agilent Semaphore"() -> (w3629:T1[])
        n1712 = local read "Previous Run Statistics"() -> (w3632:T9[])
        n1713 = local read "Disable Flood Check"() -> (w3626:bool)
        n1714 = call "WILT Station Controller.vi"("Station Number"=w3646, "GUI Aisle in"=w3648, "Drying Time (Min)"=w3630, "Current Threshold"=w3636, "Station Test State In"=w3641, "Error In"=w3645, "Aisle Location Index"=w3643, "Cool Down Period (seconds)"=w3631, "Disable Flood Check"=w3626, "Delay After Cutout (sec)"=w3628, "Previous Run Statistics"=w3632, "Send Restart Every? (Sec)"=w3633, "Agilent Valve and Switch Locations"=w3637, "Injection Times"=w3639, "Enable Start Retry"=w3635, "Day/Night Cycle"=w3638, "Final Start Presses"=w3627, "Semaphore"=w3629) -> ("GUI Aisle 1"=w3647:T3[], "Test Station Out"=w3642:T7, "Enable Start Retry Out"=w3634:bool[], "Error Out"=w3644:errorcluster)  [unwired: 5 in, 1 out]
        n1715 = Bundle By Name(cluster=w3650, "GUI Aisle 3."=w3647, "Station Test State Cluster"=w3642, "Enable Start Retry Array"=w3634) -> (w3649:T24)
        n1716 = call <vilib>:"Add State(s) to Queue__jki_lib_state_machine.vi"("State(s) in (\"\")"=w3652) -> ("States Out"=w3651:string)  [unwired: 14 in]
      }
      frame "Station 34" {
        w3670 = 1  # Aisle Location Index
        w3673 = u32 34  # Station Number
        # "Control the state of station 34"
        n1717 = Unbundle By Name(w3677) -> ("Enable Start Retry Array"=w3662:bool[], "Agilent Switches"=w3664:T2[], "GUI Aisle 3."=w3675:T3[], "Drying Time (Min)"=w3657:dbl[], "Current Threshold"=w3663:dbl, "Station Test State Cluster"=w3668:T7, "Station Timeout Values (1-56) Seconds"=w3658:dbl[], "Send Restart Every? (Sec)"=w3660:dbl, "Injection Times Input"=w3666:T15, "Day/Night Cycle Input"=w3665:T11)
        n1718 = local read "Previous Run Statistics"() -> (w3659:T9[])
        n1719 = local read "Disable Flood Check"() -> (w3653:bool)
        n1720 = local read "Delay After Cutout (Sec)"() -> (w3655:dbl)
        n1721 = local read "Final Start Presses"() -> (w3654:i32)
        n1722 = local read "Agilent Semaphore"() -> (w3656:T1[])
        n1723 = call "WILT Station Controller.vi"("Station Number"=w3673, "GUI Aisle in"=w3675, "Drying Time (Min)"=w3657, "Current Threshold"=w3663, "Station Test State In"=w3668, "Error In"=w3672, "Aisle Location Index"=w3670, "Cool Down Period (seconds)"=w3658, "Disable Flood Check"=w3653, "Delay After Cutout (sec)"=w3655, "Previous Run Statistics"=w3659, "Send Restart Every? (Sec)"=w3660, "Agilent Valve and Switch Locations"=w3664, "Injection Times"=w3666, "Enable Start Retry"=w3662, "Day/Night Cycle"=w3665, "Final Start Presses"=w3654, "Semaphore"=w3656) -> ("GUI Aisle 1"=w3674:T3[], "Test Station Out"=w3669:T7, "Enable Start Retry Out"=w3661:bool[], "Error Out"=w3671:errorcluster)  [unwired: 5 in, 1 out]
        n1724 = Bundle By Name(cluster=w3677, "GUI Aisle 3."=w3674, "Station Test State Cluster"=w3669, "Enable Start Retry Array"=w3661) -> (w3676:T24)
        n1725 = call <vilib>:"Add State(s) to Queue__jki_lib_state_machine.vi"("State(s) in (\"\")"=w3679) -> ("States Out"=w3678:string)  [unwired: 14 in]
      }
      frame "Station 35" {
        w3697 = 2  # Aisle Location Index
        w3700 = u32 35  # Station Number
        # "Control the state of station 35"
        n1726 = Unbundle By Name(w3704) -> ("Enable Start Retry Array"=w3689:bool[], "Agilent Switches"=w3691:T2[], "GUI Aisle 3."=w3702:T3[], "Drying Time (Min)"=w3684:dbl[], "Current Threshold"=w3690:dbl, "Station Test State Cluster"=w3695:T7, "Station Timeout Values (1-56) Seconds"=w3685:dbl[], "Send Restart Every? (Sec)"=w3687:dbl, "Injection Times Input"=w3693:T15, "Day/Night Cycle Input"=w3692:T11)
        n1727 = local read "Previous Run Statistics"() -> (w3686:T9[])
        n1728 = local read "Disable Flood Check"() -> (w3680:bool)
        n1729 = local read "Delay After Cutout (Sec)"() -> (w3682:dbl)
        n1730 = local read "Final Start Presses"() -> (w3681:i32)
        n1731 = local read "Agilent Semaphore"() -> (w3683:T1[])
        n1732 = call "WILT Station Controller.vi"("Station Number"=w3700, "GUI Aisle in"=w3702, "Drying Time (Min)"=w3684, "Current Threshold"=w3690, "Station Test State In"=w3695, "Error In"=w3699, "Aisle Location Index"=w3697, "Cool Down Period (seconds)"=w3685, "Disable Flood Check"=w3680, "Delay After Cutout (sec)"=w3682, "Previous Run Statistics"=w3686, "Send Restart Every? (Sec)"=w3687, "Agilent Valve and Switch Locations"=w3691, "Injection Times"=w3693, "Enable Start Retry"=w3689, "Day/Night Cycle"=w3692, "Final Start Presses"=w3681, "Semaphore"=w3683) -> ("GUI Aisle 1"=w3701:T3[], "Test Station Out"=w3696:T7, "Enable Start Retry Out"=w3688:bool[], "Error Out"=w3698:errorcluster)  [unwired: 5 in, 1 out]
        n1733 = Bundle By Name(cluster=w3704, "GUI Aisle 3."=w3701, "Station Test State Cluster"=w3696, "Enable Start Retry Array"=w3688) -> (w3703:T24)
        n1734 = call <vilib>:"Add State(s) to Queue__jki_lib_state_machine.vi"("State(s) in (\"\")"=w3706) -> ("States Out"=w3705:string)  [unwired: 14 in]
      }
      frame "Station 36" {
        w3724 = 3  # Aisle Location Index
        w3727 = u32 36  # Station Number
        # "Control the state of station 36"
        n1735 = Unbundle By Name(w3731) -> ("Enable Start Retry Array"=w3716:bool[], "Agilent Switches"=w3718:T2[], "GUI Aisle 3."=w3729:T3[], "Drying Time (Min)"=w3711:dbl[], "Current Threshold"=w3717:dbl, "Station Test State Cluster"=w3722:T7, "Station Timeout Values (1-56) Seconds"=w3712:dbl[], "Send Restart Every? (Sec)"=w3714:dbl, "Injection Times Input"=w3720:T15, "Day/Night Cycle Input"=w3719:T11)
        n1736 = local read "Previous Run Statistics"() -> (w3713:T9[])
        n1737 = local read "Disable Flood Check"() -> (w3707:bool)
        n1738 = local read "Delay After Cutout (Sec)"() -> (w3709:dbl)
        n1739 = local read "Final Start Presses"() -> (w3708:i32)
        n1740 = local read "Agilent Semaphore"() -> (w3710:T1[])
        n1741 = call "WILT Station Controller.vi"("Station Number"=w3727, "GUI Aisle in"=w3729, "Drying Time (Min)"=w3711, "Current Threshold"=w3717, "Station Test State In"=w3722, "Error In"=w3726, "Aisle Location Index"=w3724, "Cool Down Period (seconds)"=w3712, "Disable Flood Check"=w3707, "Delay After Cutout (sec)"=w3709, "Previous Run Statistics"=w3713, "Send Restart Every? (Sec)"=w3714, "Agilent Valve and Switch Locations"=w3718, "Injection Times"=w3720, "Enable Start Retry"=w3716, "Day/Night Cycle"=w3719, "Final Start Presses"=w3708, "Semaphore"=w3710) -> ("GUI Aisle 1"=w3728:T3[], "Test Station Out"=w3723:T7, "Enable Start Retry Out"=w3715:bool[], "Error Out"=w3725:errorcluster)  [unwired: 5 in, 1 out]
        n1742 = call <vilib>:"Add State(s) to Queue__jki_lib_state_machine.vi"("State(s) in (\"\")"=w3733) -> ("States Out"=w3732:string)  [unwired: 14 in]
        n1743 = Bundle By Name(cluster=w3731, "GUI Aisle 3."=w3728, "Station Test State Cluster"=w3723, "Enable Start Retry Array"=w3715) -> (w3730:T24)
      }
      frame "Station 37" {
        w3751 = 4  # Aisle Location Index
        w3754 = u32 37  # Station Number
        # "Control the state of station 37"
        n1744 = Unbundle By Name(w3758) -> ("Enable Start Retry Array"=w3743:bool[], "Agilent Switches"=w3745:T2[], "GUI Aisle 3."=w3756:T3[], "Drying Time (Min)"=w3738:dbl[], "Current Threshold"=w3744:dbl, "Station Test State Cluster"=w3749:T7, "Station Timeout Values (1-56) Seconds"=w3739:dbl[], "Send Restart Every? (Sec)"=w3741:dbl, "Injection Times Input"=w3747:T15, "Day/Night Cycle Input"=w3746:T11)
        n1745 = local read "Previous Run Statistics"() -> (w3740:T9[])
        n1746 = local read "Disable Flood Check"() -> (w3734:bool)
        n1747 = local read "Delay After Cutout (Sec)"() -> (w3736:dbl)
        n1748 = local read "Final Start Presses"() -> (w3735:i32)
        n1749 = local read "Agilent Semaphore"() -> (w3737:T1[])
        n1750 = call "WILT Station Controller.vi"("Station Number"=w3754, "GUI Aisle in"=w3756, "Drying Time (Min)"=w3738, "Current Threshold"=w3744, "Station Test State In"=w3749, "Error In"=w3753, "Aisle Location Index"=w3751, "Cool Down Period (seconds)"=w3739, "Disable Flood Check"=w3734, "Delay After Cutout (sec)"=w3736, "Previous Run Statistics"=w3740, "Send Restart Every? (Sec)"=w3741, "Agilent Valve and Switch Locations"=w3745, "Injection Times"=w3747, "Enable Start Retry"=w3743, "Day/Night Cycle"=w3746, "Final Start Presses"=w3735, "Semaphore"=w3737) -> ("GUI Aisle 1"=w3755:T3[], "Test Station Out"=w3750:T7, "Enable Start Retry Out"=w3742:bool[], "Error Out"=w3752:errorcluster)  [unwired: 5 in, 1 out]
        n1751 = Bundle By Name(cluster=w3758, "GUI Aisle 3."=w3755, "Station Test State Cluster"=w3750, "Enable Start Retry Array"=w3742) -> (w3757:T24)
        n1752 = call <vilib>:"Add State(s) to Queue__jki_lib_state_machine.vi"("State(s) in (\"\")"=w3760) -> ("States Out"=w3759:string)  [unwired: 14 in]
      }
      frame "Station 38" {
        w3778 = 5  # Aisle Location Index
        w3781 = u32 38  # Station Number
        # "Control the state of station 38"
        n1753 = Unbundle By Name(w3785) -> ("Enable Start Retry Array"=w3769:bool[], "Agilent Switches"=w3772:T2[], "GUI Aisle 3."=w3783:T3[], "Drying Time (Min)"=w3765:dbl[], "Current Threshold"=w3771:dbl, "Station Test State Cluster"=w3776:T7, "Station Timeout Values (1-56) Seconds"=w3766:dbl[], "Send Restart Every? (Sec)"=w3768:dbl, "Injection Times Input"=w3774:T15, "Day/Night Cycle Input"=w3773:T11)
        n1754 = local read "Previous Run Statistics"() -> (w3767:T9[])
        n1755 = local read "Disable Flood Check"() -> (w3761:bool)
        n1756 = local read "Delay After Cutout (Sec)"() -> (w3763:dbl)
        n1757 = local read "Final Start Presses"() -> (w3762:i32)
        n1758 = local read "Agilent Semaphore"() -> (w3764:T1[])
        n1759 = call "WILT Station Controller.vi"("Station Number"=w3781, "GUI Aisle in"=w3783, "Drying Time (Min)"=w3765, "Current Threshold"=w3771, "Station Test State In"=w3776, "Error In"=w3780, "Aisle Location Index"=w3778, "Cool Down Period (seconds)"=w3766, "Disable Flood Check"=w3761, "Delay After Cutout (sec)"=w3763, "Previous Run Statistics"=w3767, "Send Restart Every? (Sec)"=w3768, "Agilent Valve and Switch Locations"=w3772, "Injection Times"=w3774, "Enable Start Retry"=w3769, "Day/Night Cycle"=w3773, "Final Start Presses"=w3762, "Semaphore"=w3764) -> ("GUI Aisle 1"=w3782:T3[], "Test Station Out"=w3777:T7, "Enable Start Retry Out"=w3770:bool[], "Error Out"=w3779:errorcluster)  [unwired: 5 in, 1 out]
        n1760 = call <vilib>:"Add State(s) to Queue__jki_lib_state_machine.vi"("State(s) in (\"\")"=w3787) -> ("States Out"=w3786:string)  [unwired: 14 in]
        n1761 = Bundle By Name(cluster=w3785, "GUI Aisle 3."=w3782, "Station Test State Cluster"=w3777, "Enable Start Retry Array"=w3770) -> (w3784:T24)
      }
      frame "Station 39" {
        w3805 = 6  # Aisle Location Index
        w3808 = u32 39  # Station Number
        # "Control the state of station 39"
        n1762 = Unbundle By Name(w3812) -> ("Enable Start Retry Array"=w3797:bool[], "Agilent Switches"=w3799:T2[], "GUI Aisle 3."=w3810:T3[], "Drying Time (Min)"=w3792:dbl[], "Current Threshold"=w3798:dbl, "Station Test State Cluster"=w3803:T7, "Station Timeout Values (1-56) Seconds"=w3793:dbl[], "Send Restart Every? (Sec)"=w3795:dbl, "Injection Times Input"=w3801:T15, "Day/Night Cycle Input"=w3800:T11)
        n1763 = local read "Previous Run Statistics"() -> (w3794:T9[])
        n1764 = local read "Disable Flood Check"() -> (w3788:bool)
        n1765 = local read "Delay After Cutout (Sec)"() -> (w3790:dbl)
        n1766 = local read "Final Start Presses"() -> (w3789:i32)
        n1767 = local read "Agilent Semaphore"() -> (w3791:T1[])
        n1768 = call "WILT Station Controller.vi"("Station Number"=w3808, "GUI Aisle in"=w3810, "Drying Time (Min)"=w3792, "Current Threshold"=w3798, "Station Test State In"=w3803, "Error In"=w3807, "Aisle Location Index"=w3805, "Cool Down Period (seconds)"=w3793, "Disable Flood Check"=w3788, "Delay After Cutout (sec)"=w3790, "Previous Run Statistics"=w3794, "Send Restart Every? (Sec)"=w3795, "Agilent Valve and Switch Locations"=w3799, "Injection Times"=w3801, "Enable Start Retry"=w3797, "Day/Night Cycle"=w3800, "Final Start Presses"=w3789, "Semaphore"=w3791) -> ("GUI Aisle 1"=w3809:T3[], "Test Station Out"=w3804:T7, "Enable Start Retry Out"=w3796:bool[], "Error Out"=w3806:errorcluster)  [unwired: 5 in, 1 out]
        n1769 = Bundle By Name(cluster=w3812, "GUI Aisle 3."=w3809, "Station Test State Cluster"=w3804, "Enable Start Retry Array"=w3796) -> (w3811:T24)
        n1770 = call <vilib>:"Add State(s) to Queue__jki_lib_state_machine.vi"("State(s) in (\"\")"=w3814) -> ("States Out"=w3813:string)  [unwired: 14 in]
      }
      frame "Station 40" {
        w3832 = 7  # Aisle Location Index
        w3835 = u32 40  # Station Number
        # "Control the state of station 40"
        n1771 = Unbundle By Name(w3839) -> ("Enable Start Retry Array"=w3824:bool[], "Agilent Switches"=w3826:T2[], "GUI Aisle 3."=w3837:T3[], "Drying Time (Min)"=w3819:dbl[], "Current Threshold"=w3825:dbl, "Station Test State Cluster"=w3830:T7, "Station Timeout Values (1-56) Seconds"=w3820:dbl[], "Send Restart Every? (Sec)"=w3822:dbl, "Injection Times Input"=w3828:T15, "Day/Night Cycle Input"=w3827:T11)
        n1772 = local read "Delay After Cutout (Sec)"() -> (w3817:dbl)
        n1773 = local read "Final Start Presses"() -> (w3816:i32)
        n1774 = local read "Agilent Semaphore"() -> (w3818:T1[])
        n1775 = local read "Previous Run Statistics"() -> (w3821:T9[])
        n1776 = local read "Disable Flood Check"() -> (w3815:bool)
        n1777 = call "WILT Station Controller.vi"("Station Number"=w3835, "GUI Aisle in"=w3837, "Drying Time (Min)"=w3819, "Current Threshold"=w3825, "Station Test State In"=w3830, "Error In"=w3834, "Aisle Location Index"=w3832, "Cool Down Period (seconds)"=w3820, "Disable Flood Check"=w3815, "Delay After Cutout (sec)"=w3817, "Previous Run Statistics"=w3821, "Send Restart Every? (Sec)"=w3822, "Agilent Valve and Switch Locations"=w3826, "Injection Times"=w3828, "Enable Start Retry"=w3824, "Day/Night Cycle"=w3827, "Final Start Presses"=w3816, "Semaphore"=w3818) -> ("GUI Aisle 1"=w3836:T3[], "Test Station Out"=w3831:T7, "Enable Start Retry Out"=w3823:bool[], "Error Out"=w3833:errorcluster)  [unwired: 5 in, 1 out]
        n1778 = Bundle By Name(cluster=w3839, "GUI Aisle 3."=w3836, "Station Test State Cluster"=w3831, "Enable Start Retry Array"=w3823) -> (w3838:T24)
        n1779 = call <vilib>:"Add State(s) to Queue__jki_lib_state_machine.vi"("State(s) in (\"\")"=w3841) -> ("States Out"=w3840:string)  [unwired: 14 in]
      }
      frame "Station 41" {
        w3859 = 8  # Aisle Location Index
        w3862 = u32 41  # Station Number
        # "Control the state of station 41"
        n1780 = Unbundle By Name(w3866) -> ("Enable Start Retry Array"=w3850:bool[], "Agilent Switches"=w3853:T2[], "GUI Aisle 3."=w3864:T3[], "Drying Time (Min)"=w3846:dbl[], "Current Threshold"=w3852:dbl, "Station Test State Cluster"=w3857:T7, "Station Timeout Values (1-56) Seconds"=w3847:dbl[], "Send Restart Every? (Sec)"=w3849:dbl, "Injection Times Input"=w3855:T15, "Day/Night Cycle Input"=w3854:T11)
        n1781 = local read "Delay After Cutout (Sec)"() -> (w3844:dbl)
        n1782 = local read "Final Start Presses"() -> (w3843:i32)
        n1783 = local read "Agilent Semaphore"() -> (w3845:T1[])
        n1784 = local read "Previous Run Statistics"() -> (w3848:T9[])
        n1785 = local read "Disable Flood Check"() -> (w3842:bool)
